vi "AWG_Main.vi"() -> ()   [LabVIEW 2016, in "ZI AWG.lvlib"]
doc: "Control a Zurich instrument device via the LabOne Labview API. \nRequirements: Zurich Instruments UHFLI \nThis example shows how to start a AWG module and measure it with the scope module.\n\n© Zurich Instruments AG, www.zhinst.com"
uses:
  ZI AWG.lvlib
  Ctl_SetParameter(Value).ctl
  <instrlib>/Zurich Instruments LabOne/Zurich Instruments LabOne.lvlib
  General.lvlib
panel:
  out "Error Out":errorcluster
  in  "Address":string="DEV8029"
  out "Selected Device":string
  # "const pulse_zeros_head_samples = 1000;\nconst pulse_zeros_tail_samples = 1;\nconst pulse_ones_samples = 500000;\n\nwave wave_pulse_zeros_head = zeros(pulse_zeros_head_samples);\nwave wave_pulse_zeros_tail = zeros(pulse_zeros_tail_samples);\n// wave wave_pulse_ones = ones(pulse_ones_samples);\nwave wave_pulse_ones = gauss(pulse_ones_samples, 1, pulse_ones_samples/2, pulse_ones_samples/6);\n\nwave wave_pulse = join(wave_pulse_zeros_head, wave_pulse_ones, wave_pulse_zeros_tail);\n\nwhile (true){\n  waitDigTrigger(1);\n  setTrigger(0b1111);\n  playWave(wave_pulse);\n  waitWave();\n  setTrigger(0b0000);\n}"
  # "ziExample-UHFLI-Module-AWGvi\nRequirements: UHFLI\nsee block diagram for VI description"
  # "Tested Devices:\n- HDAWG"
  # "const pulse_zeros_head_samples = 1000;\nconst pulse_zeros_tail_samples = 1;\nconst pulse_ones_samples = 500000;\n\nwave wave_pulse_zeros_head = zeros(pulse_zeros_head_samples);\nwave wave_pulse_zeros_tail = zeros(pulse_zeros_tail_samples);\nwave wave_pulse_ones = ones(pulse_ones_samples);\n\nwave wave_pulse = join(wave_pulse_zeros_head, wave_pulse_ones, wave_pulse_zeros_tail);\n\nwhile (true){\n  waitDigTrigger(1);\n  setTrigger(0b1111);\n  playWave(wave_pulse);\n  waitWave();\n  setTrigger(0b0000);\n}"
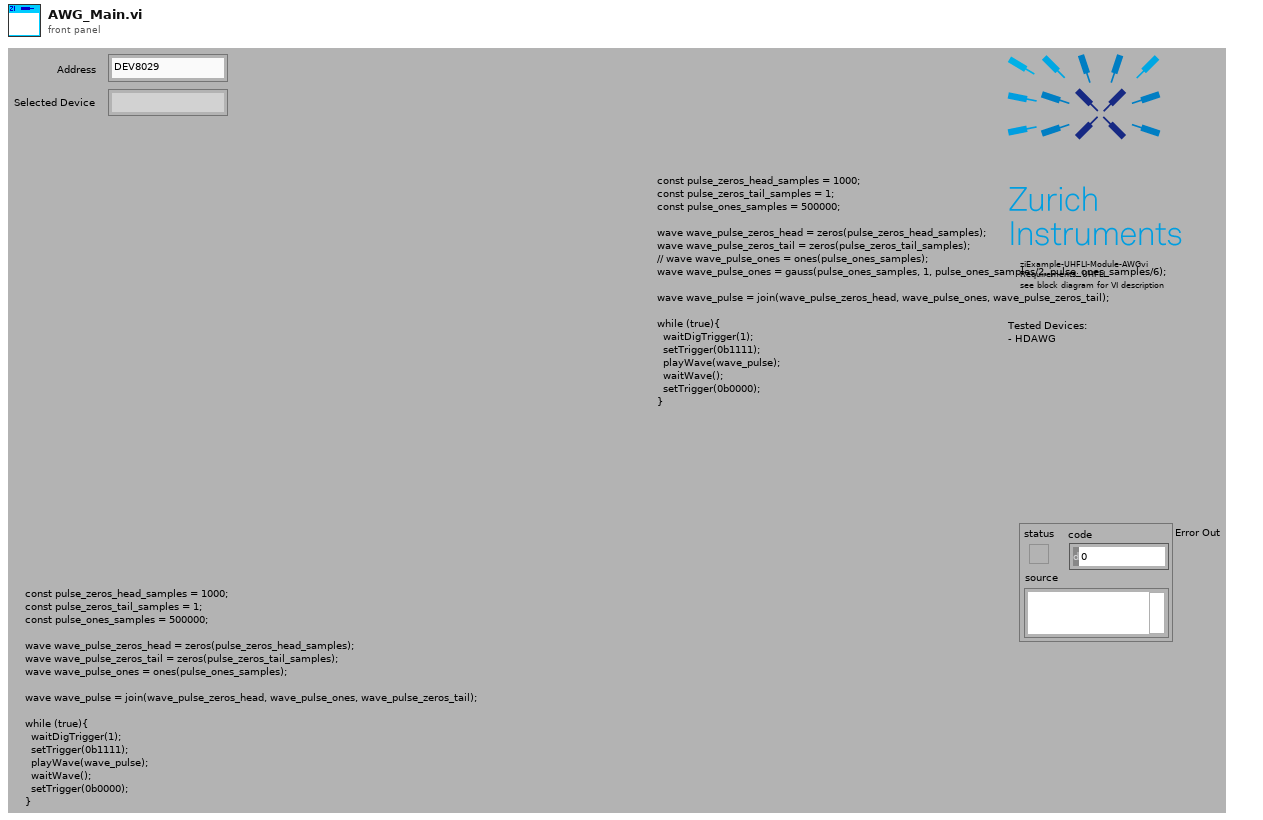
[diagram p1: front panel]
types:
  T1 = typedef "General.lvlib/Ctl_SetParameter(Value).ctl" = cluster{"Path":string, "Value":dbl, "comment":string}
  T2 = typedef "Zurich Instruments LabOne.lvlib/ziTypeHandle.ctl" = cluster{"handleValid":bool, "Conn":u64, "Path Prefix":string, "Handle":u64, "Connected":bool, "Clockbase(s)":dbl}
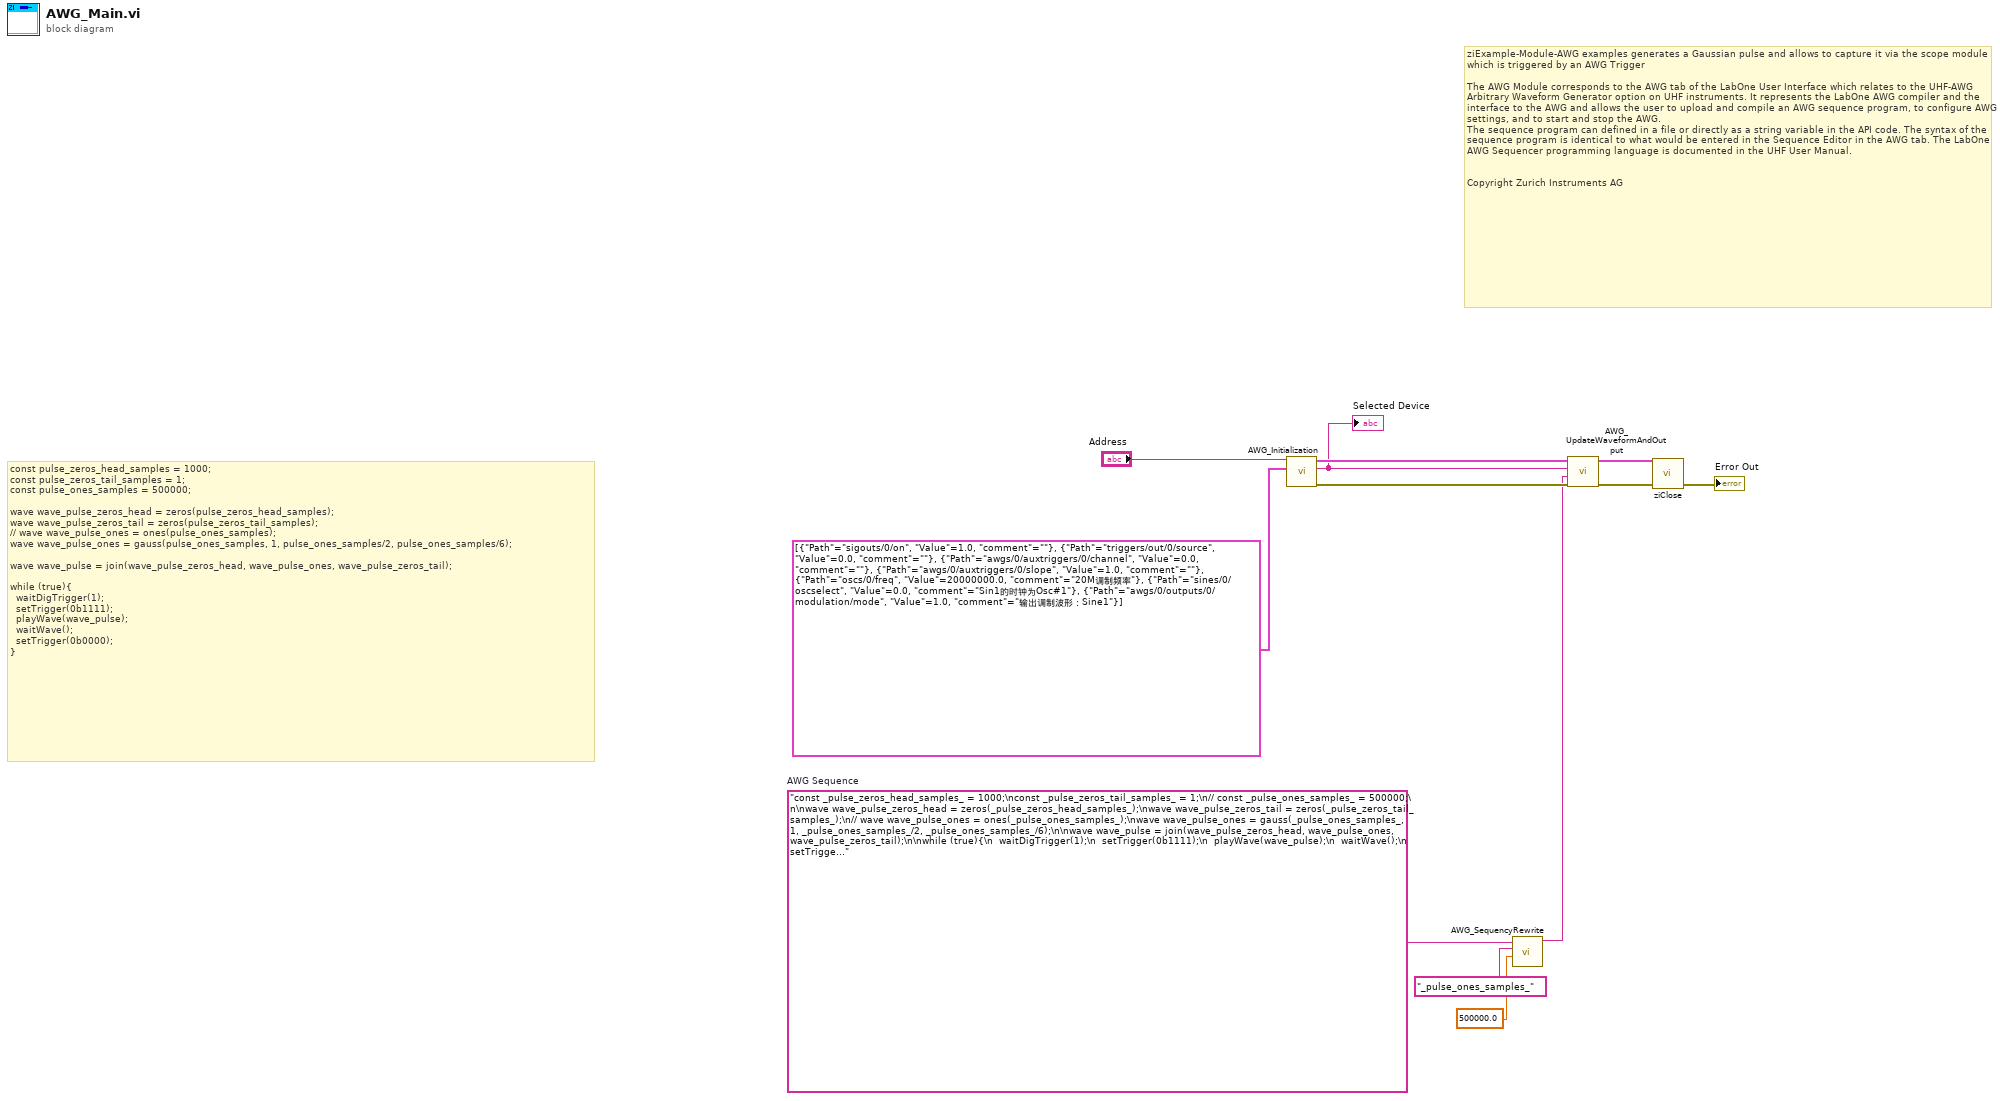
[diagram p0: block diagram]
diagram:
  w3 = "const _pulse_zeros_head_samples_ = 1000;\nconst _pulse_zeros_tail_samples_ = 1;\n// const _pulse_ones_samples_ = 500000;\n\nwave wave_pulse_zeros_head = zeros(_pulse_zeros_head_samples_);\nwave wave_pulse_zeros_tail = zeros(_pulse_zeros_tail_samples_);\n// wave wave_pulse_ones = ones(_pulse_ones_samples_);\nwave wave_pulse_ones = gauss(_pulse_ones_samples_, 1, _pulse_ones_samples_/2, _pulse_ones_samples_/6);\n\nwave wave_pulse = join(wave_pulse_zeros_head, wave_pulse_ones, wave_pulse_zeros_tail);\n\nwhile (true){\n  waitDigTrigger(1);\n  setTrigger(0b1111);\n  playWave(wave_pulse);\n  waitWave();\n  setTrigger(0b0000);\n}"  # AWG Sequence
  # "const pulse_zeros_head_samples = 1000;\nconst pulse_zeros_tail_samples = 1;\nconst pulse_ones_samples = 500000;\n\nwave wave_pulse_zeros_head = zeros(pulse_zeros_head_samples);\nwave wave_pulse_zeros_tail = zeros(pulse_zeros_tail_samples);\n// wave wave_pulse_ones = ones(pulse_ones_samples);\nwave wave_pulse_ones = gauss(pulse_ones_samples, 1, pulse_ones_samples/2, pulse_ones_samples/6);\n\nwave wave_pulse = join(wave_pulse_zeros_head, wave_pulse_ones, wave_pulse_zeros_tail);\n\nwhile (true){\n  waitDigTrigger(1);\n  setTrigger(0b1111);\n  playWave(wave_pulse);\n  waitWave();\n  setTrigger(0b0000);\n}"
  # "ziExample-Module-AWG examples generates a Gaussian pulse and allows to capture it via the scope module which is triggered by an AWG Trigger\n\nThe AWG Module corresponds to the AWG tab of the LabOne User Interface which relates to the UHF-AWG Arbitrary Waveform Generator option on UHF instruments. It represents the LabOne AWG compiler and the interface to the AWG and allows the user to upload and compile an AWG sequence program, to configure AWG settings, and to start and stop the AWG.\nThe sequence program can defined in a file or directly as a string variable in the API code. The syntax of the sequence program is identical to what would be entered in the Sequence Editor in the AWG tab. The LabOne AWG Sequencer programming language is documented in the UHF User Manual.\n\n\nCopyright Zurich Instruments AG"
  n1 = call "AWG_Initialization.vi"("AWG Parameters"=T1[] [{"Path"="sigouts/0/on", "Value"=1.0, "comment"=""}, {"Path"="triggers/out/0/source", "Value"=0.0, "comment"=""}, {"Path"="awgs/0/auxtriggers/0/channel", "Value"=0.0, "comment"=""}, {"Path"="awgs/0/auxtriggers/0/slope", "Value"=1.0, "comment"=""}, {"Path"="oscs/0/freq", "Value"=20000000.0, "comment"="20M调制频率"}, {"Path"="sines/0/oscselect", "Value"=0.0, "comment"="Sin1的时钟为Osc#1"}, {"Path"="awgs/0/outputs/0/modulation/mode", "Value"=1.0, "comment"="输出调制波形：Sine1"}] ("Parameters"), "Address"="Address") -> ("error out"=w8:errorcluster, "Selected Device"=w7:string, "AWG Handle Out"=w9:T2)  [unwired: 7 in]
  "Selected Device" <- w7
  n2 = call "AWG_SequencyRewrite.vi"("Value"=500000.0, "Constant Name"="_pulse_ones_samples_", "AWG Sequence"=w3) -> ("result string"=w4:string)  [unwired: 6 in, 2 out]
  n3 = call "AWG_UpdateWaveformAndOutput.vi"("Error In"=w8, "AWG Sequence"=w4, "Selected Device"=w7, "AWG Handle In"=w9) -> ("error out"=w5:errorcluster, "AWG Handle Out"=w6:T2)  [unwired: 6 in]
  n4 = call <instrlib>:"ziClose.vi"("Error In"=w5, "Handle In"=w6) -> ("Error Out"=→"Error Out":errorcluster)  [unwired: 2 in, 1 out]
